vi "Find all memory hogs in memory.vi"() -> ()   [LabVIEW 2013]
doc: "This .vi searches all .vi's in memory and returns a list sorted by the amount memory they are using. This .vi is helpful to find .vis that have stored large amounts of data on the diagram or in the default values."
panel:
  out "memory sum (k)":dbl=91.2412109375
  out "total # of .vis":i32=1
  out "Array":cluster{"Metric.DataSize":u32, "Name":string}[](array[cluster])
  out "Total # standard .vis":i32
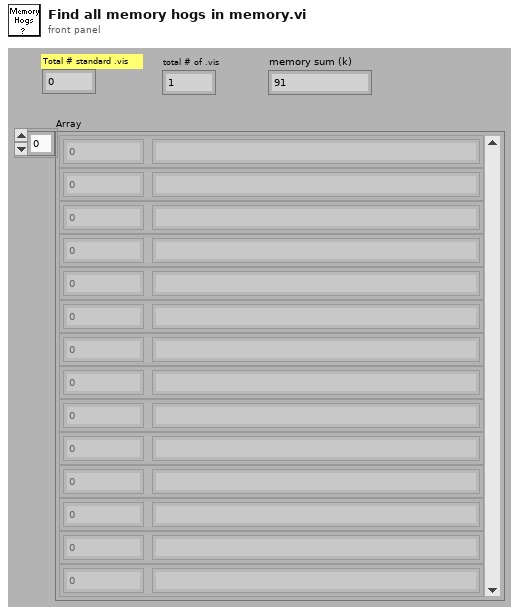
[diagram p1: front panel]
types:
  T1 = enum32{"invalid VI type", "Standard VI", "Control VI", "Global VI", "Polymorphic VI", "Configuration VI", "SubSystem", "Facade VI", "Method VI", "Statechart Diagram VI"}
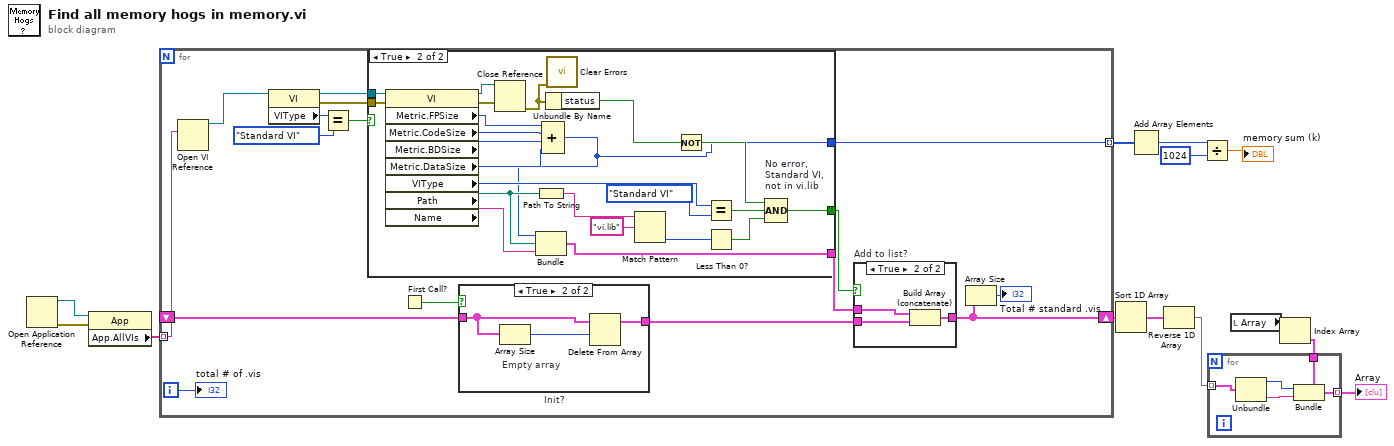
[diagram p0: block diagram]
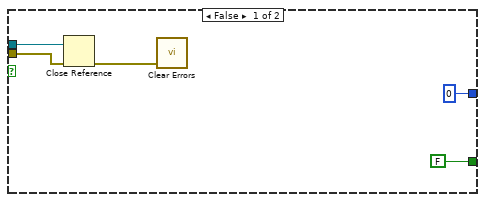
[diagram p2: hidden frame]
diagram:
  n1 = Open Application Reference() -> (0:w9:errorcluster, 3:w13:refnum<vi>)  [unwired: 1 in, 3 out]
  n2 = property class="App"(reference=w13, error in=w9) -> ("App.AllVIs"=w12:string[])  [unwired: 2 out]
  n3 = for {
    tunnel: w12 -> [w29] mode=indexing
    shift-right: [w21] -> w11
    shift-left: _ -> [w27]
    tunnel: [w20] -> w6 mode=indexing
    i -> [w23]
    n4 = Open VI Reference(vi path=w29) -> (vi reference=w19:refnum<vi>)  [unwired: 1 in, 5 out]
    n5 = property class="VI"(reference=w19) -> (reference out=w18:refnum<vi>, error out=w17:errorcluster, "VIType"=w15:T1)  [unwired: 1 in]
    n6 = Equal?(x=w15, y=T1."Standard VI" ("VI Type")) -> (x = y?=w14:bool)
    n7 = case shown="True" w14 {
      tunnel: [_ w49] -> w28
      tunnel: [FALSE w48] -> w24
      tunnel: [u32 0 w37] -> w20
      tunnel: w18 -> [w32 w36]
      tunnel: w17 -> [w31 w35]
      frame False {
        n8 = Close Reference(reference=w32, error in (no error)=w31) -> (error out=w30:errorcluster)
        n9 = call <vilib>:"Clear Errors.vi"("error in (no error)"=w30) -> ()  [unwired: 7 out]
      }
      frame True {
        n10 = property class="VI"(reference=w36, error in=w35) -> (reference out=w40:refnum<vi>, error out=w41:errorcluster, "Metric.FPSize"=w38:u32, "Metric.CodeSize"=w42:u32, "Metric.BDSize"=w43:u32, "Metric.DataSize"=w44:u32, "VIType"=w57:T1, "Path"=w51:path, "Name"=w50:string)
        n11 = Close Reference(reference=w40, error in (no error)=w41) -> (error out=w39:errorcluster)
        n12 = Path To String(path=w51) -> (string=w52:string)
        n13 = Compound Arithmetic op=ADD(w38, w42, w43, w44) -> (w37:u32)
        n14 = Bundle(w37, "Path"=w51, "Name"=w50) -> (w49:cluster{u32, "Path":path, "Name":string})  [unwired: 1 out]
        n15 = Unbundle By Name(w39) -> ("status"=w46:bool)
        n16 = call <vilib>:"Clear Errors.vi"("error in (no error)"=w39) -> ()  [unwired: 7 out]
        n17 = Match Pattern(string=w52, regular expression="vi.lib") -> (offset past match=w54:i32)  [unwired: 4 out]
        n18 = Not(x=w46) -> (.not. x?=w45:bool)
        n19 = Equal?(x=w57, y=T1."Standard VI" ("VI Type")) -> (x = y?=w47:bool)
        n20 = Less Than 0?(x=w54) -> (x < 0?=w53:bool)
        n21 = Compound Arithmetic op=AND "No error,\nStandard VI,\nnot in vi.lib"(w45, w47, w53) -> (w48:bool)
      }
    }
    n22 = First Call?() -> (First Call?: T/F=w25:bool)
    n23 = case "Init?" shown="True" w25 {
      tunnel: w27 -> [w58 w61]
      tunnel: [w58 w59] -> w26
      frame False {
      }
      frame True {
        # "Empty array"
        n24 = Array Size(array=w61) -> (size(s)=w60:i32)
        n25 = Delete From Array(array=w61, length=w60) -> (array with subset deleted=w59:cluster{u32, "Path":path, "Name":string}[])  [unwired: 1 in, 1 out]
      }
    }
    n26 = case "Add to list?" shown="True" w24 {
      tunnel: w26 -> [w62 w65]
      tunnel: [w62 w64] -> w21
      tunnel: w28 -> [_ w63]
      frame False {
      }
      frame True {
        n27 = Build Array (concatenate)(w63, w65) -> (w64:cluster{u32, "Path":path, "Name":string}[])
      }
    }
    n28 = Array Size(array=w21) -> (size(s)=→"Total # standard .vis":i32)
    "total # of .vis" <- w23
  }
  n29 = Sort 1D Array(array=w11) -> (sorted array=w10:cluster{u32, "Path":path, "Name":string}[])
  n30 = Add Array Elements(numeric array=w6) -> (sum=w5:u32)
  n31 = Reverse 1D Array(array=w10) -> (reversed array=w7:cluster{u32, "Path":path, "Name":string}[])
  n32 = Divide(x=w5, y=u32 1024) -> (x/y=→"memory sum (k)":dbl)
  n33 = local read "Array"() -> (w2:cluster{"Metric.DataSize":u32, "Name":string}[])
  n34 = Index Array(array=w2) -> (element=w1:cluster{"Metric.DataSize":u32, "Name":string})  [unwired: 1 in]
  n35 = for {
    tunnel: w7 -> [w70] mode=indexing
    tunnel: [w67] -> w8 mode=indexing
    tunnel: w1 -> [w66]
    n36 = Unbundle(w70) -> (w69:u32, "Name"=w68:string)  [unwired: 1 out]
    n37 = Bundle(cluster=w66, "Metric.DataSize"=w69, "Name"=w68) -> (w67:cluster{"Metric.DataSize":u32, "Name":string})
  }
  "Array" <- w8
